vi "__Test.vi"() -> ()   [LabVIEW 2019, in "CAN-NI.lvlib"]
uses:
  CAN-NI.lvlib
  CAN-Interface/TypeDef/Def-CANData.ctl
  CAN-NI.lvclass
  CAN-Interface/TypeDef/Def-PreConfig-BaudRate.ctl
  CAN-Interface/TypeDef/Def-BaudRate.ctl
  CAN-Interface/TypeDef/Def-PreConfig-Termination.ctl
  CAN-Interface/TypeDef/Def-Termination.ctl
  CAN-Interface/TypeDef/Def-ReceiveData.ctl
  CAN-Interface/TypeDef/Def-TransmitData.ctl
  CAN-Interface/TypeDef/Def-PayLoad.ctl
  CAN-Interface/Class-Interface.lvclass
panel:
  out "FrameData":T1
  out "error out":errorcluster
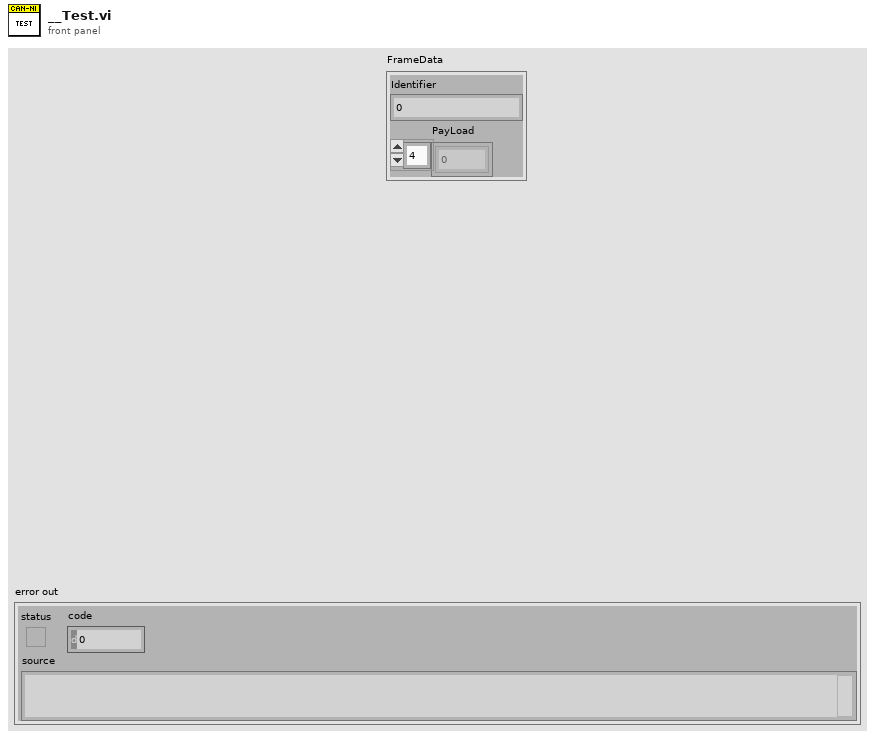
[diagram p1: front panel]
types:
  T1 = typedef "CAN-Interface.lvlib/Class-Interface.lvclass/Def-CANData.ctl" = cluster{"Identifier":u32, "PayLoad":u8[]}
  T2 = typedef "CAN-Interface.lvlib/Class-Interface.lvclass/Def-ReceiveData.ctl" = cluster{"Channel Num":u32, "timeout(ms)":i32}
  T3 = typedef "CAN-Interface.lvlib/Class-Interface.lvclass/Def-PreConfig-Termination.ctl" = cluster{"Channel Num":u32, "Termination":T4}
  T4 = typedef "CAN-Interface.lvlib/Class-Interface.lvclass/Def-Termination.ctl" = enum8{"on", "off"}
  T5 = typedef "CAN-Interface.lvlib/Class-Interface.lvclass/Def-PreConfig-BaudRate.ctl" = cluster{"Channel Num":u32, "BaudRate":T6}
  T6 = typedef "CAN-Interface.lvlib/Class-Interface.lvclass/Def-BaudRate.ctl" = u32
  T7 = typedef "CAN-Interface.lvlib/Class-Interface.lvclass/Def-TransmitData.ctl" = cluster{"Channel Num":u32, "Frame":cluster{"Identifier":u32, "PayLoad":T8}}
  T8 = typedef "CAN-Interface.lvlib/Class-Interface.lvclass/Def-PayLoad.ctl" = cluster{"byte1":u8, "byte2":u8, "byte3":u8, "byte4":u8, "byte5":u8, "byte6":u8, "byte7":u8, "byte8":u8}
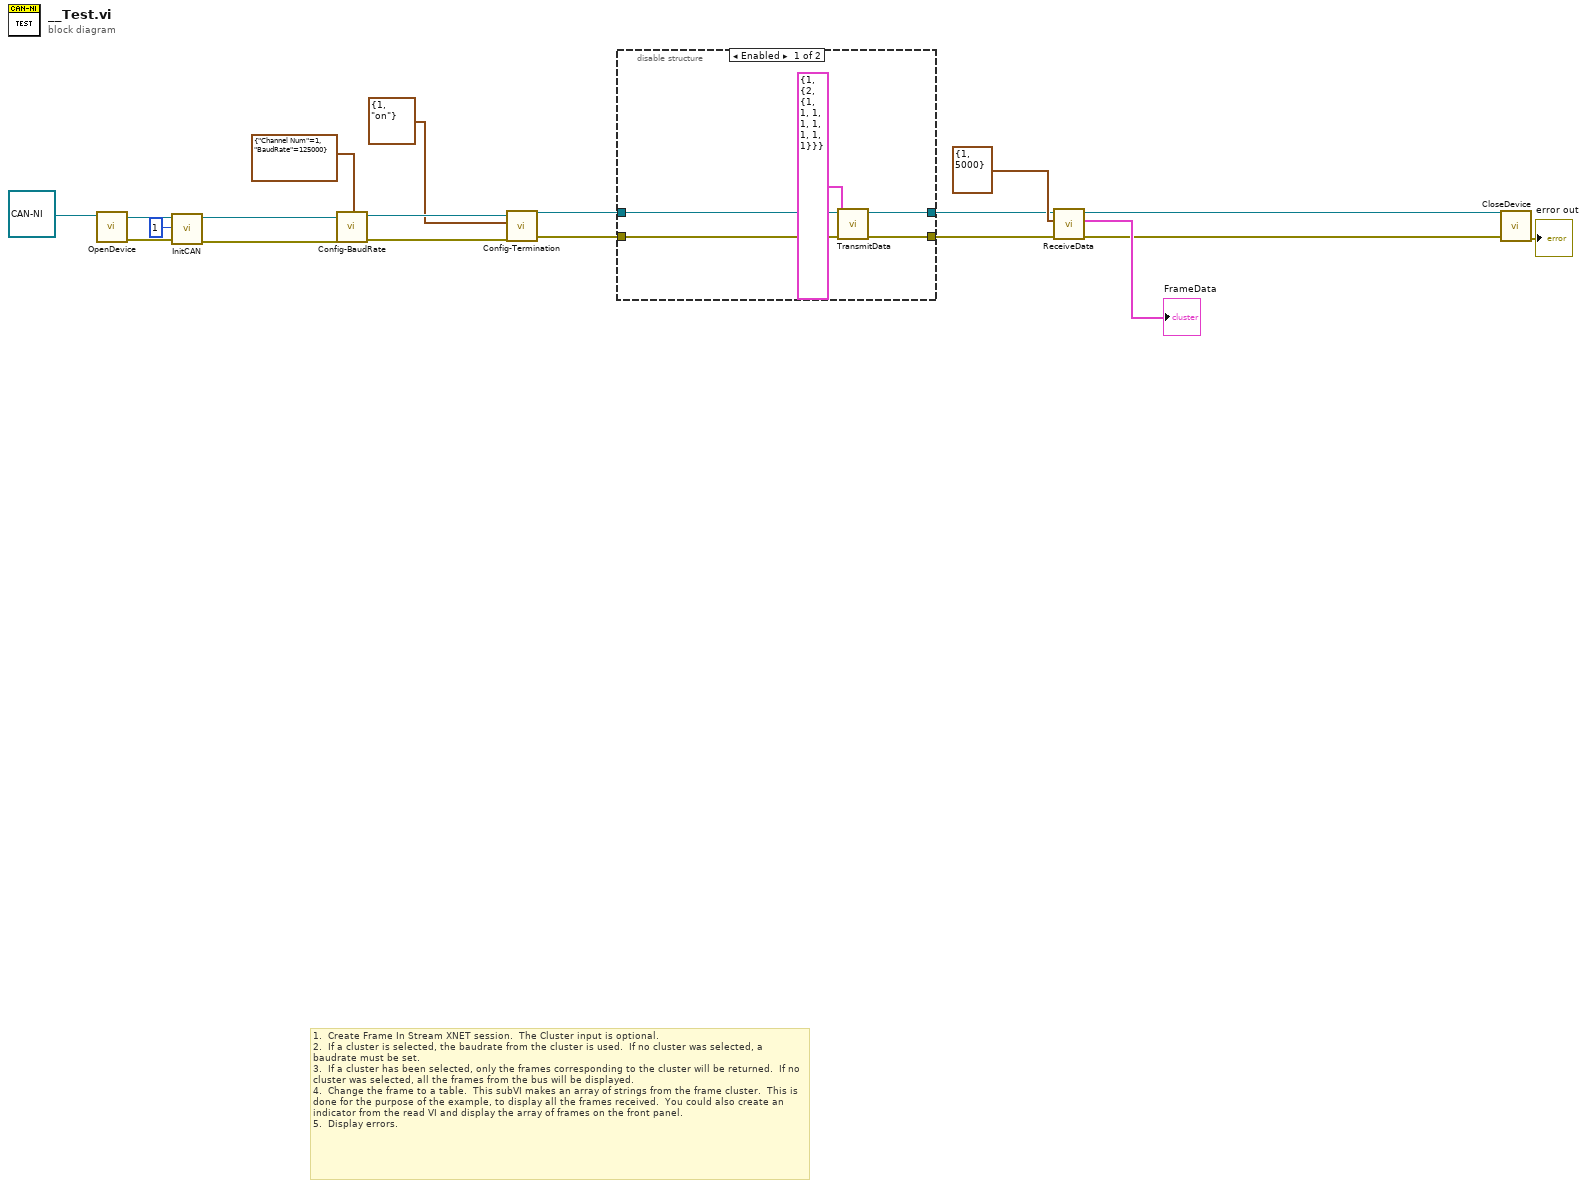
[diagram p0: block diagram]
diagram:
  # "1.  Create Frame In Stream XNET session.  The Cluster input is optional.  \n2.  If a cluster is selected, the baudrate from the cluster is used.  If no cluster was selected, a baudrate must be set.\n3.  If a cluster has been selected, only the frames corresponding to the cluster will be returned.  If no cluster was selected, all the frames from the bus will be displayed.\n4.  Change the frame to a table.  This subVI makes an array of strings from the frame cluster.  This is done for the purpose of the example, to display all the frames received.  You could also create an indicator from the read VI and display the array of frames on the front panel. \n5.  Display errors."
  n1 = call-dynamic "OpenDevice.vi"("CAN-NI in"=refnum<class "CAN-NI.lvclass"> refnum ("CAN-NI.lvlib:CAN-NI.lvclass")) -> ("error out"=w19:errorcluster, "CAN-NI out"=w16:refnum<class "CAN-NI.lvclass">)  [unwired: 9 in]
  n2 = call-dynamic "InitCAN.vi"("error in (no error)"=w19, "Channel Num"=u32 1, "CAN-NI in"=w16) -> ("error out"=w12:errorcluster, "CAN-NI out"=w14:refnum<class "CAN-NI.lvclass">)  [unwired: 7 in]
  n3 = call-dynamic "Config-BaudRate.vi"("error in (no error)"=w12, "Def-PreConfig-BaudRate"=T5 {"Channel Num"=1, "BaudRate"=125000}, "CAN-NI in"=w14) -> ("error out"=w9:errorcluster, "CAN-NI out"=w10:refnum<class "CAN-NI.lvclass">)  [unwired: 7 in]
  n4 = call-dynamic "Config-Termination.vi"("error in (no error)"=w9, "Def-PreConfig-Termination"=T3 {"Channel Num"=1, "Termination"=enum."on"}, "CAN-NI in"=w10) -> ("error out"=w6:errorcluster, "CAN-NI out"=w7:refnum<class "CAN-NI.lvclass">)  [unwired: 7 in]
  n5 = disable-structure shown="Enabled" {
    disable-tunnel: w7 -> [w24 w26]
    disable-tunnel: w6 -> [w23 w25]
    disable-tunnel: [w22 w26] -> w2
    disable-tunnel: [w21 w25] -> w1
    frame Enabled {
      n6 = call-dynamic "TransmitData.vi"("error in (no error)"=w23, "Def-TransmitData"=T7 {"Channel Num"=1, "Frame"={"Identifier"=2, "PayLoad"={"byte1"=1, "byte2"=1, "byte3"=1, "byte4"=1, "byte5"=1, "byte6"=1, "byte7"=1, "byte8"=1}}}, "CAN-NI in"=w24) -> ("error out"=w21:errorcluster, "CAN-NI out"=w22:refnum<class "CAN-NI.lvclass">)  [unwired: 7 in]
    }
    frame Disabled {
    }
  }
  n7 = call-dynamic "ReceiveData.vi"("error in (no error)"=w1, "Def-ReceiveData"=T2 {"Channel Num"=1, "timeout(ms)"=5000}, "CAN-NI in"=w2) -> ("error out"=w3:errorcluster, "FrameData"=→"FrameData":T1, "CAN-NI out"=w15:refnum<class "CAN-NI.lvclass">)  [unwired: 6 in]
  n8 = call-dynamic "CloseDevice.vi"("error in (no error)"=w3, "CAN-NI in"=w15) -> ("error out"=→"error out":errorcluster)  [unwired: 8 in, 1 out]
